vi "FCI Bin Test_EON.vi"(8 "error in (no error)":errorcluster, 11 "Image 3":T1) -> (0 "error IO":errorcluster, 2 "EON outer width":sgl format="%.2f")   [LabVIEW 2019, in "Algorithm.lvclass"]
uses:
  FrameworkOverrides/Algorithm.lvclass
  <vilib>/vision/NI_Vision_Development_Module.lvlib
  <vilib>/vision/Measure.llb/Straight Edge Process.ctl
  <vilib>/vision/Measure.llb/Straight Edge Options.ctl
  <vilib>/vision/Measure.llb/Edge Polarity.ctl
  <vilib>/vision/Measure.llb/Edge Options.ctl
  <vilib>/vision/Image Controls.llb/IMAQ Image.ctl
panel:
  out "x-y":u32
  out "ROI Descriptor":T2 {"Contours"."Type" items=["No Selection", "Point", "Line", "Rectangle", "Oval", "Polygon", "Freehand Region", "Annulus", "Unused2", "Unused3", "Broken Line", "Freehand Line", "Rotated Rectangle"]}
  out "EON Presence/Absence":bool
  out "Angle (Pixel)":dbl
  in  "Y coord lower limit":dbl=350.0 format="%#_13g"
  in  "Y coord upper limit":dbl=730.0 format="%#_13g"
  out "Y Coord":dbl[](array[numeric])
  out "Number of Particles":i32
  out "subarray 2":dbl[](array[numeric])
  out "index of element":i32
  out "Array":bool[](array[boolean])
  out "X Coord":dbl[](array[numeric])
  out "Image 2":T1(plugin-control)
  out "Image":T1(plugin-control)
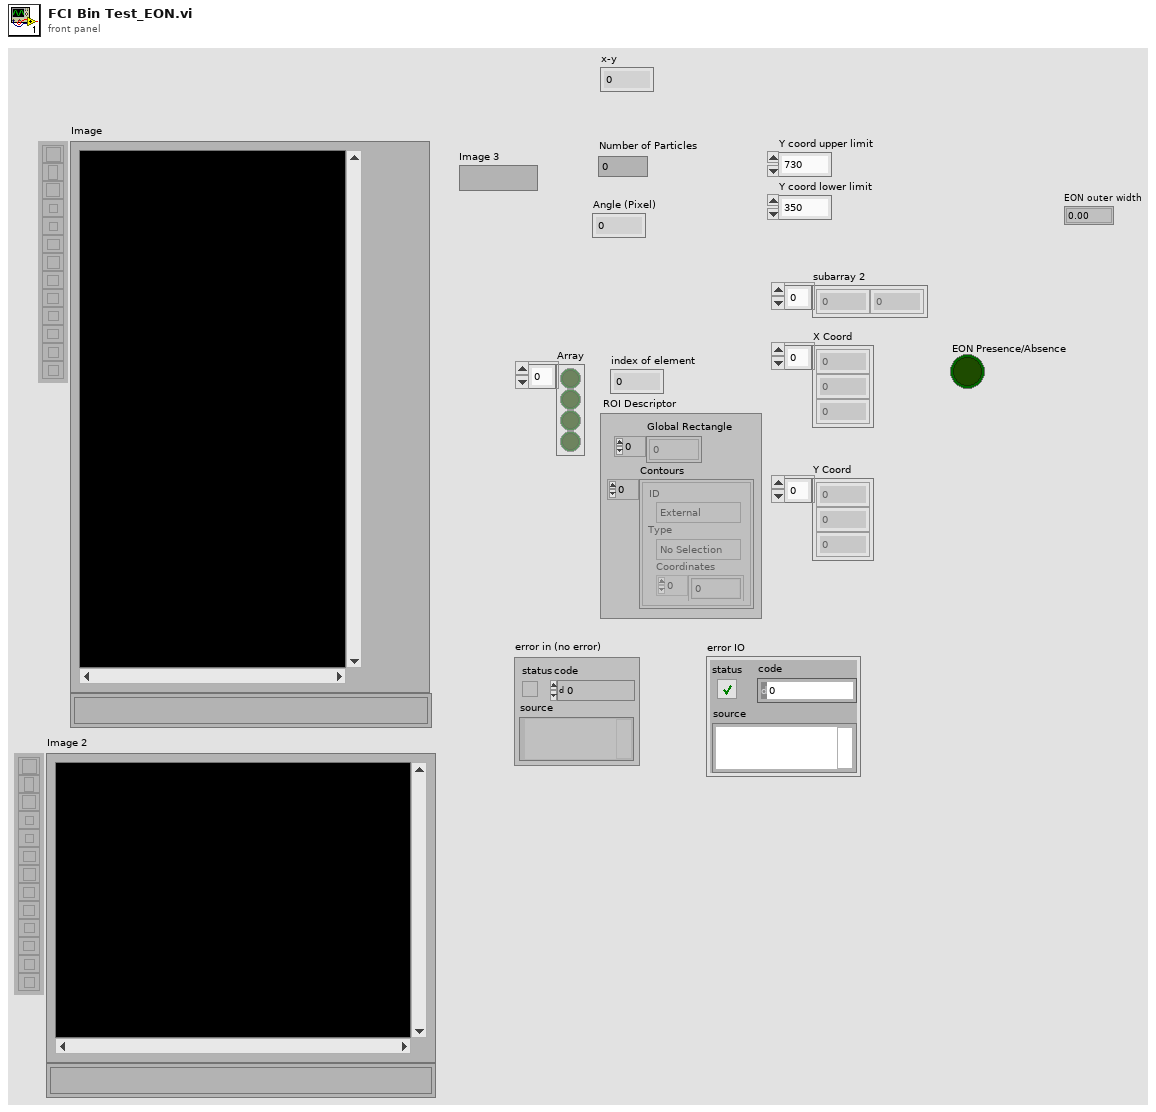
[diagram p1: front panel]
types:
  T1 = typedef "IMAQ Image.ctl" = refnum<image>
  T2 = typedef "ROI Descriptor" = cluster{"Global Rectangle":i32[], "Contours":cluster{"ID":enum32{"External", "Internal"}, "Type":u32, "Coordinates":i32[]}[]}
  T3 = typedef "Edge Options.ctl" = cluster{"Edge Polarity":T4, "Kernel Size":u32, "Width":u32, "Minimum Edge Strength":sgl, "Interpolation Type":enum32{"Zero Order", "Bilinear", "Quadratic", "Cubic", "Bilinear Fixed"}, "Data Processing Method":enum32{"Average", "Median"}}
  T4 = typedef "Edge Polarity.ctl" = u32
  T5 = cluster{"Search Direction":u32, "Edge Options":T3, "Show Search Area":bool, "Show Search Lines":bool, "Show Edges Found":bool, "Show Result":bool, "Search Area Color":u32, "Search Lines Color":u32, "Edge Locations Color":u32, "Result Color":u32, "Overlay Group Name":string}
  T6 = typedef "Straight Edge Options.ctl" = cluster{"Number of Lines":i32, "Type":T7, "Min. Score":dbl, "Max. Score":dbl, "Orientation":dbl, "Angle Range":dbl, "Angle Tolerance":dbl, "Step Size":u32, "Min. SNR (db)":dbl, "Min. Points (%)":dbl, "Hough Iterations":i32}
  T7 = typedef "Straight Edge Process.ctl" = enum32{"First Edge Rake", "Best Edge Rake", "Hough Edge Rake", "First Edge Projection", "Best Edge Projection"}
  T8 = cluster{"Left":dbl, "Top":dbl, "Right":dbl, "Bottom":dbl, "Angle":dbl}
  T9 = typedef "Particle Parameters" = i32
  T10 = cluster{"Measurement Parameter":T9, "Range Lower Value":dbl, "Range Upper Value":dbl, "Range":bool, "Measurement Type":bool}[]
  T11 = typedef "Image Type" = u32
  T12 = cluster{"Point1 (Pixels)":cluster{"X":sgl, "Y":sgl}, "Point2 (Pixels)":cluster{"X":sgl, "Y":sgl}, "Point1 (Real-World)":cluster{"X":sgl, "Y":sgl}, "Point2 (Real-World)":cluster{"X":sgl, "Y":sgl}, "Angle (Pixel)":dbl, "Angle (Real-World)":dbl, "Score":dbl, "Straightness":dbl, "Average SNR (db)":dbl, "Calibration Valid":bool}[]
  T13 = cluster{"Point1 (Pixels)":cluster{"X":sgl, "Y":sgl}, "Point2 (Pixels)":cluster{"X":sgl, "Y":sgl}, "Point1 (Real-World)":cluster{"X":sgl, "Y":sgl}, "Point2 (Real-World)":cluster{"X":sgl, "Y":sgl}, "Angle (Pixel)":dbl, "Angle (Real-World)":dbl, "Score":dbl, "Straightness":dbl, "Average SNR (db)":dbl, "Calibration Valid":bool}
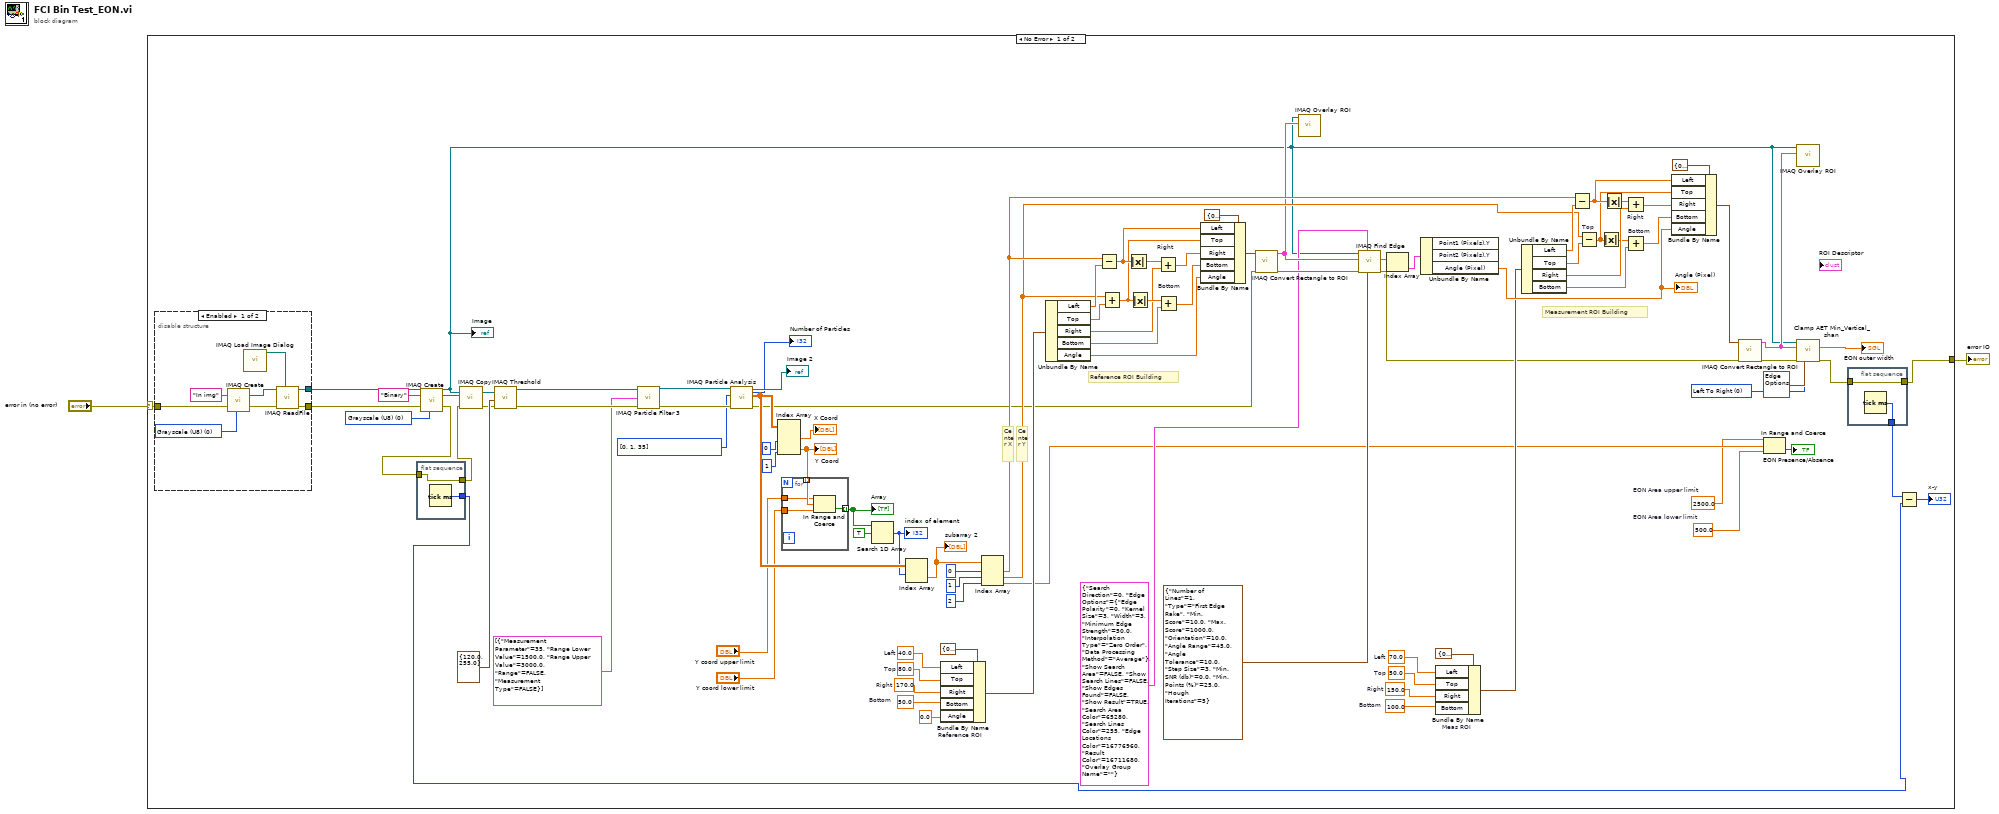
[diagram p0: block diagram]
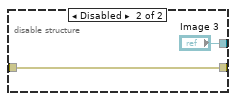
[diagram p2: hidden frame]
diagram:
  n1 = case shown="No Error" "error in (no error)" {
    selector: "error in (no error)" -> [w24 w117]
    tunnel: [w6 w117] -> w1
    frame No Error {
      w10 = u16 0 items=["Left To Right", "Right To Left", "Top To Bottom", "Bottom To Top"] ("Scanning axis")
      w19 = 500.0  # EON Area lower limit
      w20 = 2500.0  # EON Area upper limit
      w32 = 100.0  # Bottom
      w33 = 150.0  # Right
      w34 = 50.0  # Top
      w35 = 70.0  # Left
      w39 = 50.0  # Bottom
      w40 = 170.0  # Right
      w41 = 80.0  # Top
      w42 = 40.0  # Left
      w91 = T9[] [0, 1, 35] items=["Center of Mass X", "Center of Mass Y", "First Pixel X", "First Pixel Y", "Bounding Rect Left", "Bounding Rect Top", "Bounding Rect Right", "Bounding Rect Bottom", "Max Feret Diameter Start X", "Max Feret Diameter Start Y", "Max Feret Diameter End X", "Max Feret Diameter End Y", "Max Horiz. Segment Length Left", "Max Horiz. Segment Length Right", "Max Horiz. Segment Length Row", "-", "Bounding Rect Width", "Bounding Rect Height", "Bounding Rect Diagonal", "Perimeter", "Convex Hull Perimeter", "Holes' Perimeter", "Max Feret Diameter", "Equivalent Ellipse Major Axis", "Equivalent Ellipse Minor Axis", "Equivalent Ellipse Minor Axis (Feret)", "Equivalent Rect Long Side", "Equivalent Rect Short Side", "Equivalent Rect Diagonal", "Equivalent Rect Short Side (Feret)", "Average Horiz. Segment Length", "Average Vert. Segment Length", "Hydraulic Radius", "Waddel Disk Diameter", "-", "Area", "Holes' Area", "Particle & Holes' Area", "Convex Hull Area", "Image Area", "-", "Number of Holes", "Number of Horiz. Segments", "Number of Vert. Segments", "-", "Orientation", "Max Feret Diameter Orientation", "-", "% Area/Image Area", "% Area/(Particle & Holes' Area)", "Ratio of Equivalent Ellipse Axes", "Ratio of Equivalent Rect Sides", "-", "Elongation Factor", "Compactness Factor", "Heywood Circularity Factor", "Type Factor", "-", "Sum X", "Sum Y", "Sum XX", "Sum XY", "Sum YY", "Sum XXX", "Sum XXY", "Sum XYY", "Sum YYY", "-", "Moment of Inertia XX", "Moment of Inertia XY", "Moment of Inertia YY", "Moment of Inertia XXX", "Moment of Inertia XXY", "Moment of Inertia XYY", "Moment of Inertia YYY", "Norm. Moment of Inertia XX", "Norm. Moment of Inertia XY", "Norm. Moment of Inertia YY", "Norm. Moment of Inertia XXX", "Norm. Moment of Inertia XXY", "Norm. Moment of Inertia XYY", "Norm. Moment of Inertia YYY", "Hu Moment 1", "Hu Moment 2", "Hu Moment 3", "Hu Moment 4", "Hu Moment 5", "Hu Moment 6", "Hu Moment 7"] ("Pixel Measurements")
      w97 = T11 0 items=["Grayscale (U8)", "Grayscale (I16)", "Grayscale (SGL)", "Complex (CSG)", "RGB (U32)", "HSL (U32)", "RGB (U64)", "Grayscale (U16)"] ("Image Type")
      # "Measurement ROI Building"
      # "Reference ROI Building"
      # "Center Y"
      # "Center X"
      n2 = disable-structure shown="Enabled" {
        disable-tunnel: [w102 w108] -> w61
        disable-tunnel: w24 -> [w100 w108]
        disable-tunnel: [w99 "Image 3"] -> w11
        frame Enabled {
          w104 = T11 0 items=["Grayscale (U8)", "Grayscale (I16)", "Grayscale (SGL)", "Complex (CSG)", "RGB (U32)", "HSL (U32)", "RGB (U64)", "Grayscale (U16)"] ("Image Type")
          n3 = call "IMAQ Create"("Image Name"="In img", "Image Type"=w104, "error in (no error)"=w100) -> ("New Image"=w106:T1, "error out"=w103:errorcluster)  [unwired: 2 in]
          n4 = call "IMAQ Load Image Dialog"() -> ("Path"=w101:path)  [unwired: 9 in, 2 out]
          n5 = call "IMAQ ReadFile"("File Path"=w101, "error in (no error)"=w103, "Image"=w106) -> ("error out"=w102:errorcluster, "Image Out"=w99:T1)  [unwired: 4 in, 3 out]
        }
        frame Disabled {
        }
      }
      "Image" <- w11
      n6 = flat-sequence {
        tunnel: w9 -> [w112]
        tunnel: [w112] -> w8
        tunnel: [w111] -> w4
        frame #0 {
          n7 = Tick Count (ms)() -> (millisecond timer value=w111:u32)
        }
      }
      n8 = call "IMAQ Create"("Image Name"="Binary", "Image Type"=w97, "error in (no error)"=w61) -> ("New Image"=w96:T1, "error out"=w9:errorcluster)  [unwired: 2 in]
      n9 = call "IMAQ Copy"("error in (no error)"=w8, "Image Dst"=w96, "Image Src"=w11) -> ("error out"=w26:errorcluster, "Image Dst Out"=w62:T1)  [unwired: 3 in]
      n10 = call "IMAQ Threshold"("error in (no error)"=w26, "Range"=cluster{"Lower value":sgl, "Upper value":sgl} {"Lower value"=120.0, "Upper value"=255.0}, "Image Src"=w62) -> ("error out"=w95:errorcluster, "Image Dst Out"=w94:T1)  [unwired: 7 in]
      n11 = call "IMAQ Particle Filter 3"("Image Src"=w94, "Selection Values"=T10 [{"Measurement Parameter"=35, "Range Lower Value"=1500.0, "Range Upper Value"=3000.0, "Range"=FALSE, "Measurement Type"=FALSE}], "error in (no error)"=w95) -> ("Image Dst Out"=w93:T1, "error out"=w92:errorcluster)  [unwired: 10 in, 1 out]
      n12 = call "IMAQ Particle Analysis"("error in (no error)"=w92, "Pixel Measurements"=w91, "Image"=w93) -> ("error out"=w25:errorcluster, "Particle Measurements (Pixels)"=w57:dbl[][], "Image Out (duplicate)"=→"Image 2":T1, "Number of Particles"=→"Number of Particles":i32)  [unwired: 3 in, 2 out]
      n13 = Index Array(array=w57, index (col) #1=0 ("disabled index (col)"), index (col) #2=1 ("index (col)")) -> (element #1=→"X Coord":dbl[], element #2=w48:dbl[])  [unwired: 2 in]
      "Y Coord" <- w48
      n14 = for {
        tunnel: w48 -> [w116] mode=indexing
        tunnel: [w115] -> w59 mode=indexing
        tunnel: "Y coord upper limit" -> [w114]
        tunnel: "Y coord lower limit" -> [w113]
        n15 = In Range and Coerce(upper limit=w114, x=w116, lower limit=w113) -> (In Range?=w115:bool)  [unwired: 1 out]
      }
      "Array" <- w59
      n16 = Search 1D Array(1D array=w59, element=TRUE) -> (index of element=w56:i32)  [unwired: 1 in]
      "index of element" <- w56
      n17 = Index Array(array=w57, index (row)=w56) -> (element=w55:dbl[])  [unwired: 1 in]
      "subarray 2" <- w55
      n18 = Bundle By Name "Reference ROI"(cluster=T8 {"Left"=0.0, "Top"=0.0, "Right"=0.0, "Bottom"=0.0, "Angle"=0.0} ("input cluster"), "Left"=w42, "Top"=w41, "Right"=w40, "Bottom"=w39, "Angle"=0.0) -> (w36:T8)
      n19 = Index Array(array=w55, index #1=0 ("index"), index #2=1 ("index"), index #3=2 ("index")) -> (element #1=w52:dbl, element #2=w43:dbl, element #3=w21:dbl)
      n20 = Unbundle By Name(w36) -> ("Left"=w74:dbl, "Top"=w73:dbl, "Right"=w72:dbl, "Bottom"=w71:dbl, "Angle"=w70:dbl)
      n21 = Subtract(x=w52, y=w74) -> (x-y=w82:dbl)
      n22 = Add(x=w43, y=w73) -> (x+y=w81:dbl)
      n23 = Absolute Value(x=w82) -> (abs(x)=w85:dbl)
      n24 = Absolute Value(x=w81) -> (abs(x)=w84:dbl)
      n25 = Add "Right"(x=w85, y=w72) -> (x+y=w80:dbl)
      n26 = Add "Bottom"(x=w84, y=w71) -> (x+y=w79:dbl)
      n27 = Bundle By Name(cluster=T8 {"Left"=0.0, "Top"=0.0, "Right"=0.0, "Bottom"=0.0, "Angle"=0.0} ("input cluster"), "Left"=w82, "Top"=w81, "Right"=w80, "Bottom"=w79, "Angle"=w70) -> (w64:T8)
      n28 = call "IMAQ Convert Rectangle to ROI"("error in (no error)"=w25, "Rectangle"=w64) -> ("error out"=w69:errorcluster, "ROI Descriptor"=w29:T2)  [unwired: 7 in]
      n29 = call "IMAQ Overlay ROI"("ROI Descriptor"=w29, "Image"=w11) -> ()  [unwired: 8 in, 2 out]
      n30 = call "IMAQ Find Edge"("Line Fit Options"=T6 {"Number of Lines"=1, "Type"=enum."First Edge Rake", "Min. Score"=10.0, "Max. Score"=1000.0, "Orientation"=10.0, "Angle Range"=45.0, "Angle Tolerance"=10.0, "Step Size"=3, "Min. SNR (db)"=0.0, "Min. Points (%)"=25.0, "Hough Iterations"=5}, "Options"=T5 {"Search Direction"=0, "Edge Options"={"Edge Polarity"=0, "Kernel Size"=3, "Width"=3, "Minimum Edge Strength"=50.0, "Interpolation Type"=enum."Zero Order", "Data Processing Method"=enum."Average"}, "Show Search Area"=FALSE, "Show Search Lines"=FALSE, "Show Edges Found"=FALSE, "Show Result"=TRUE, "Search Area Color"=65280, "Search Lines Color"=255, "Edge Locations Color"=16776960, "Result Color"=16711680, "Overlay Group Name"=""}, "error in (no error)"=w69, "ROI Descriptor"=w29, "Image"=w11) -> ("error out"=w14:errorcluster, "Straight Edges"=w67:T12)  [unwired: 3 in, 2 out]
      n31 = Index Array(array=w67) -> (element=w66:T13)  [unwired: 1 in]
      n32 = Unbundle By Name(w66) -> ("Angle (Pixel)"=w65:dbl)  [unwired: 2 out]
      "Angle (Pixel)" <- w65
      n33 = Bundle By Name "Meas ROI"(cluster=T8 {"Left"=0.0, "Top"=0.0, "Right"=0.0, "Bottom"=0.0, "Angle"=0.0} ("input cluster"), "Left"=w35, "Top"=w34, "Right"=w33, "Bottom"=w32) -> (w30:T8)
      n34 = Unbundle By Name(w30) -> ("Left"=w78:dbl, "Top"=w77:dbl, "Right"=w76:dbl, "Bottom"=w75:dbl)
      n35 = Subtract(x=w52, y=w78) -> (x-y=w88:dbl)
      n36 = Subtract "Top"(x=w43, y=w77) -> (x-y=w44:dbl)
      n37 = Absolute Value(x=w44) -> (abs(x)=w45:dbl)
      n38 = Absolute Value(x=w88) -> (abs(x)=w90:dbl)
      n39 = Add "Right"(x=w90, y=w76) -> (x+y=w87:dbl)
      n40 = Add "Bottom"(x=w45, y=w75) -> (x+y=w86:dbl)
      n41 = Bundle By Name(cluster=T8 {"Left"=0.0, "Top"=0.0, "Right"=0.0, "Bottom"=0.0, "Angle"=0.0} ("input cluster"), "Left"=w88, "Top"=w44, "Right"=w87, "Bottom"=w86, "Angle"=w65) -> (w15:T8)
      n42 = call "IMAQ Convert Rectangle to ROI"("error in (no error)"=w14, "Rectangle"=w15) -> ("error out"=w13:errorcluster, "ROI Descriptor"=w12:T2)  [unwired: 7 in]
      n43 = In Range and Coerce(upper limit=w20, x=w21, lower limit=w19) -> (In Range?=→"EON Presence/Absence":bool)  [unwired: 1 out]
      n44 = call "IMAQ Overlay ROI"("ROI Descriptor"=w12, "Image"=w11) -> ()  [unwired: 8 in, 2 out]
      n45 = call "Clamp AET Min_Vertical_shan.vi"("Image"=w11, "Scanning axis"=w10, "ROI Descriptor"=w12, "error in (no error)"=w13, "Edge Options"=T3 {"Edge Polarity"=0, "Kernel Size"=3, "Width"=3, "Minimum Edge Strength"=50.0, "Interpolation Type"=enum."Zero Order", "Data Processing Method"=enum."Average"}) -> ("Distance"=→"EON outer width":sgl, "error out"=w7:errorcluster)  [unwired: 4 in, 5 out]
      n46 = flat-sequence {
        tunnel: w7 -> [w110]
        tunnel: [w110] -> w6
        tunnel: [w109] -> w5
        frame #0 {
          n47 = Tick Count (ms)() -> (millisecond timer value=w109:u32)
        }
      }
      n48 = Subtract(x=w5, y=w4) -> (x-y=→"x-y":u32)
    }
    frame Error {
    }
  }
  "error IO" <- w1
